vi "save channels to raw bin files.vi"(6 "T:galvo F:resonant default:T":bool=TRUE, 8 "frame number in":i32, 9 "last frame":bool, 10 "image data in (SGL)":sgl[][](array[numeric]), 11 "image data in (U16)":u16[][](array[numeric])) -> ()   [LabVIEW 2012]
doc: "SciScan 1.0 151216"
uses:
  Custom Controls/file format type def.ctl
  GFG/GFGpathGet.vi
  GFG/GFG library.lvlib
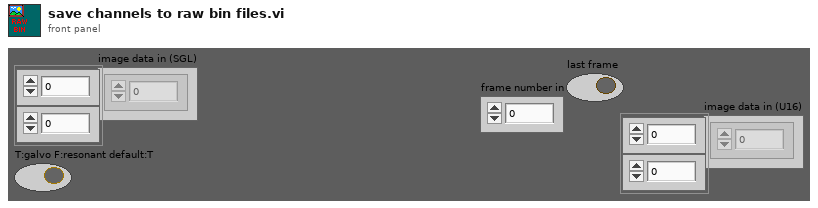
[diagram p1: front panel]
types:
  T1 = enum16{"open", "replace", "create", "open or create", "replace or create", "replace or create with confirmation"}
  T2 = typedef "file format type def.ctl" = enum16{"16bit raw", "32bit raw", "16bit multi-tiff (interleave)", "16bit multi-tiff (separate)", "16bit multi-tiff (stacked)", "32bit multi-tiff (interleave)", "32bit multi-tiff (separate)", "32bit multi-tiff (stacked)", "16bit tiff series (interleave)", "16bit tiff series (separate)", "16bit tiff series (stacked)", "32bit tiff series (interleave)", "32bit tiff series (separate)", "32bit tiff series (stacked)"}
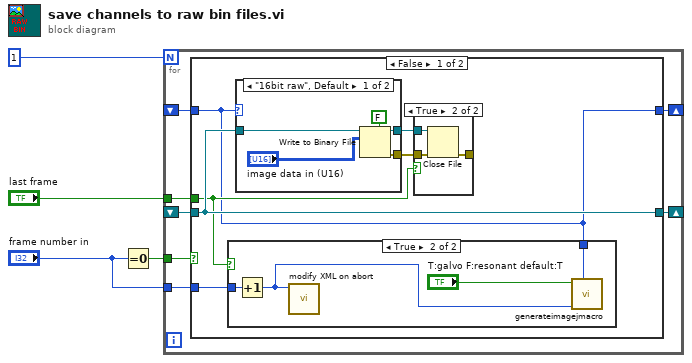
[diagram p0: block diagram]
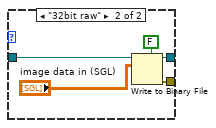
[diagram p4: hidden frame]
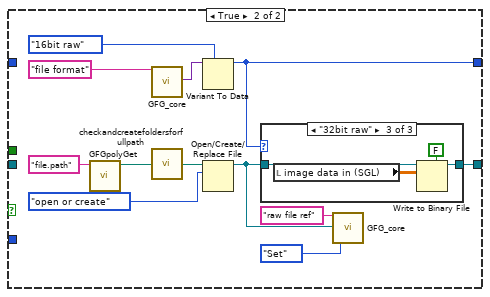
[diagram p5: hidden frame]
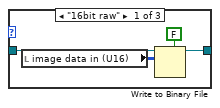
[diagram p6: hidden frame]
diagram:
  n1 = Equal To 0?(x="frame number in") -> (x = 0?=w3:bool)
  n2 = for {
    N: 1 -> [_]
    tunnel: w3 -> [w11]
    shift-right: [w10] -> _
    shift-left: _ -> [w9]
    shift-right: [w8] -> _
    shift-left: _ -> [w7]
    tunnel: "last frame" -> [w6]
    tunnel: "frame number in" -> [w5]
    n3 = case shown="False" w11 {
      tunnel: w7 -> [w12 _]
      tunnel: [w15 w39] -> w10
      tunnel: w9 -> [w15 _]
      tunnel: [w12 w44] -> w8
      tunnel: w6 -> [w14 _]
      tunnel: w5 -> [w13 _]
      frame False {
        n4 = case shown="True" w14 {
          tunnel: w13 -> [_ w20]
          tunnel: w12 -> [_ w19]
          frame False {
          }
          frame True {
            n5 = Increment(x=w20) -> (x+1=w18:i32)
            n6 = call "modify XML on abort.vi"("frame number"=w18) -> ()  [unwired: 10 in, 1 out]
            n7 = call "generateimagejmacro.vi"("file format"=w19, "number of recorded frames"=w18, "Reso or Galvo?"="T:galvo F:resonant default:T") -> ()  [unwired: 9 in]
          }
        }
        n8 = case shown="\"16bit raw\", Default" w12 {
          tunnel: w15 -> [w29 w34]
          tunnel: [w28 w33] -> w16
          tunnel: [w27 w32] -> w17
          frame "16bit raw", Default {
            n9 = Write to Binary File(file (use dialog)=w29, data="image data in (U16)", 5:FALSE ("prepend array or string size? (T)")) -> (refnum out=w27:refnum<file>, error out=w28:errorcluster)  [unwired: 3 in, 1 out]
          }
          frame "32bit raw" {
            n10 = Write to Binary File(file (use dialog)=w34, data="image data in (SGL)", 5:FALSE ("prepend array or string size? (T)")) -> (refnum out=w32:refnum<file>, error out=w33:errorcluster)  [unwired: 3 in, 1 out]
          }
        }
        n11 = case shown="True" w14 {
          tunnel: w17 -> [_ w25]
          tunnel: w16 -> [w22 w24]
          tunnel: [w22 w23] -> _
          frame False {
          }
          frame True {
            n12 = Close File(refnum=w25, error in=w24) -> (error out=w23:errorcluster)  [unwired: 1 out]
          }
        }
      }
      frame True {
        n13 = call-poly "GFGpolyGet.vi"("Variable Name in"="file.path") -> ("Path"=w42:path)  [unwired: 8 in, 2 out]
        n14 = call "GFG_core.vi"("Variable Name in"="file format") -> ("Variant Out"=w46:variant)  [unwired: 12 in, 6 out]
        n15 = call "checkandcreatefoldersforfullpath.vi"("Path IN"=w42) -> ("Path OUT"=w41:path)  [unwired: 4 in]
        n16 = Variant To Data(type=file_format_type_def."16bit raw" ("file format"), Variant=w46) -> (data=w44:T2)  [unwired: 1 in, 1 out]
        n17 = Open/Create/Replace File(file path (use dialog)=w41, operation (0:open)=T1."open or create") -> (refnum out=w38:refnum<file>)  [unwired: 4 in, 2 out]
        n18 = case shown="\"32bit raw\"" w44 {
          tunnel: w38 -> [w50 w52 w55]
          tunnel: [w49 w52 w54] -> w39
          frame "16bit raw" {
            n19 = local read "image data in (U16)"() -> (w48:u16[][])
            n20 = Write to Binary File(file (use dialog)=w50, data=w48, 5:FALSE ("prepend array or string size? (T)")) -> (refnum out=w49:refnum<file>)  [unwired: 3 in, 2 out]
          }
          frame Default {
          }
          frame "32bit raw" {
            n21 = local read "image data in (SGL)"() -> (w53:sgl[][])
            n22 = Write to Binary File(file (use dialog)=w55, data=w53, 5:FALSE ("prepend array or string size? (T)")) -> (refnum out=w54:refnum<file>)  [unwired: 3 in, 2 out]
          }
        }
        n23 = call "GFG_core.vi"("Variable Name in"="raw file ref", "Variant in"=w38, "Action"=enum16{"Init", "Set", "Get", "Clear"}."Set") -> ()  [unwired: 10 in, 7 out]
      }
    }
  }
